vi "Configure Limit Test Auto Clear.vi"(0 "VISA resource name":refnum<visa-resource-name>, 5 "Limit Test Number (1)":u16=1, 7 "Enable Auto Clear (ON)":bool=TRUE, 9 "Function (0: Volts)":u16(ring) items=["Volts", "Current", "Resistance", "Digitize Voltage", "Digitize Current"], 11 "error in (no error)":errorcluster) -> (4 "VISA resource name out":refnum<visa-resource-name>, 15 "error out":errorcluster)   [LabVIEW 2020, in "Keithley 2450.lvlib"]
doc: "Configures limit testing settings, such as the source of the tested value, binning, and I/O settings."
uses:
  Keithley 2450.lvlib
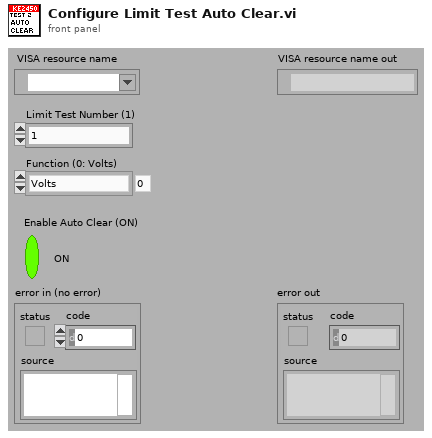
[diagram p1: front panel]
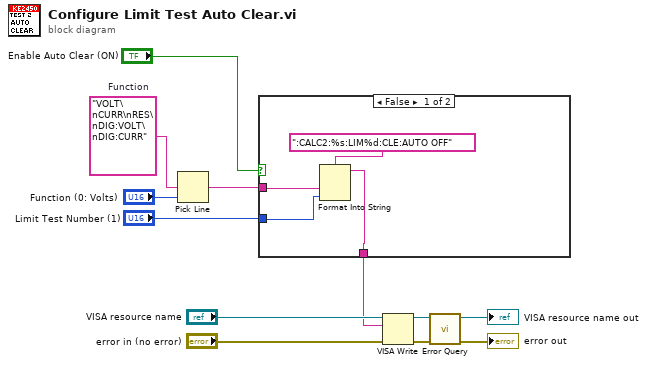
[diagram p0: block diagram]
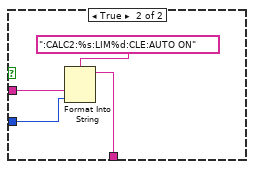
[diagram p2: hidden frame]
diagram:
  w5 = "VOLT\nCURR\nRES\nDIG:VOLT\nDIG:CURR"  # Function
  n1 = Pick Line(multi-line string=w5, line index="Function (0: Volts)") -> (output string=w3:string)  [unwired: 1 out]
  n2 = case shown="False" "Enable Auto Clear (ON)" {
    tunnel: [w13 w19] -> w6
    tunnel: w3 -> [w15 w18]
    tunnel: "Limit Test Number (1)" -> [w14 w17]
    frame False {
      n3 = Format Into String(format string=":CALC2:%s:LIM%d:CLE:AUTO OFF", w15, w14) -> (resulting string=w13:string)  [unwired: 2 in, 1 out]
    }
    frame True {
      n4 = Format Into String(format string=":CALC2:%s:LIM%d:CLE:AUTO ON", w18, w17) -> (resulting string=w19:string)  [unwired: 2 in, 1 out]
    }
  }
  n5 = VISA Write(VISA resource name="VISA resource name", write buffer=w6, error in (no error)="error in (no error)") -> (VISA resource name out=w8:refnum<visa-resource-name>, error out=w7:errorcluster)  [unwired: 1 out]
  n6 = call "Error Query.vi"("error in (no error)"=w7, "VISA resource name"=w8) -> ("error out"=→"error out":errorcluster, "VISA resource name out"=→"VISA resource name out":refnum<visa-resource-name>)  [unwired: 8 out]
